vi "ke2002_init.vi"(8 "error in":errorcluster, 11 "VISA in":refnum<visa-resource-name>) -> (0 "error out":errorcluster, 2 "ID":string, 3 "VISA out":refnum<visa-resource-name>)   [LabVIEW 2020]
uses:
  <vilib>/Instr/_visa.llb/VISA GPIB Control REN Mode.ctl
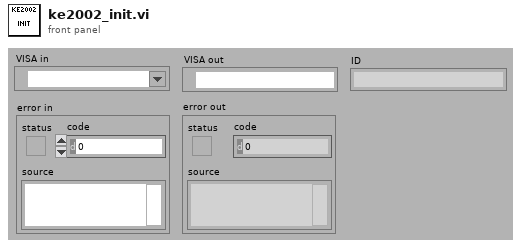
[diagram p1: front panel]
types:
  T1 = cluster{"Status":bool, "Code":i32, "Source (VI Name)":string}
  T2 = cluster{"error":bool, "code":i32, "source":string}
  T3 = typedef "VISA GPIB Control REN Mode.ctl" = u16
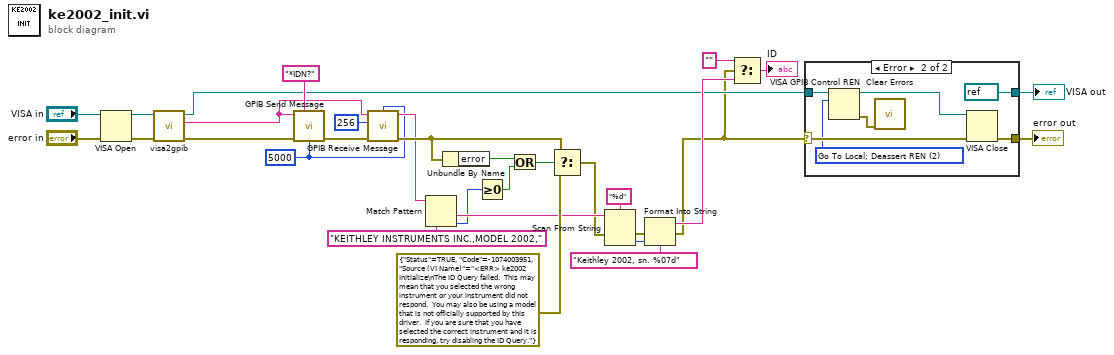
[diagram p0: block diagram]
diagram:
  w1 = u32 5000 ("timeout ms")
  n1 = VISA Open(error in (no error)="error in", VISA resource name="VISA in") -> (VISA resource name=w25:refnum<visa-resource-name>, error out=w26:errorcluster)  [unwired: 3 in]
  n2 = call "visa2gpib.vi"("error in"=w26, "VISA in"=w25) -> ("error out"=w24:errorcluster, "combined address"=w23:string, "VISA out"=w4:refnum<visa-resource-name>)  [unwired: 7 in]
  n3 = call "GPIB Send Message.vi"("timeout ms"=w1, "address string"=w23, "write buffer"="*IDN?", "error in"=w24) -> ("error out"=w31:T2)  [unwired: 3 in, 2 out]
  n4 = call "GPIB Receive Message.vi"("timeout ms"=w1, "address string"=w23, "byte count"=256, "error in"=w31) -> ("read buffer"=w17:string, "error out"=w19:T2)  [unwired: 3 in, 1 out]
  n5 = Match Pattern(string=w17, regular expression="KEITHLEY INSTRUMENTS INC.,MODEL 2002,") -> (after substring=w16:string, offset past match=w7:i32)  [unwired: 1 in, 2 out]
  n6 = Unbundle By Name(w19) -> ("error"=w21:bool)
  n7 = Greater Or Equal To 0?(x=w7) -> (x >= 0?=w6:bool)
  n8 = Or(x=w21, y=w6) -> (x .or. y?=w22:bool)
  n9 = Select(t=w19, s=w22, f=T1 {"Status"=TRUE, "Code"=-1074003951, "Source (VI Name)"="<ERR> ke2002 Initialize\nThe ID Query failed.  This may mean that you selected the wrong instrument or your instrument did not respond.  You may also be using a model that is not officially supported by this driver.  If you are sure that you have selected the correct instrument and it is responding, try disabling the ID Query."}) -> (s? t:f=w14:T1)
  n10 = Scan From String(format string="%d", input string=w16, error in=w14) -> (error out=w13:errorcluster, output 1=w12:i32)  [unwired: 2 in, 2 out]
  n11 = Format Into String(format string="Keithley 2002, sn. %07d", error in=w13, w12) -> (resulting string=w10:string, error out=w2:errorcluster)  [unwired: 1 in]
  n12 = Select(t="", s=w2, f=w10) -> (s? t:f=→"ID":string)
  n13 = case shown="Error" w2 {
    selector: w2 -> [w32 w38]
    tunnel: [w32 w40] -> w5
    tunnel: w4 -> [w33 w37]
    tunnel: [w33 refnum<visa-resource-name> refnum ("VISA out")] -> w3
    frame No Error {
    }
    frame Error {
      w35 = T3 2 items=["Deassert REN", "Assert REN", "Go To Local; Deassert REN ", "Assert REN; Address Device", "Local Lockout (Addressed Devices)", "Local Lockout (This Device)", "Go To Local"] ("Mode")
      n14 = VISA GPIB Control REN(10:w35, 11:w37) -> (0:w34:errorcluster, 3:w36:refnum<visa-resource-name>)  [unwired: 1 in]
      n15 = call <vilib>:"Clear Errors.vi"("error in (no error)"=w34) -> ()  [unwired: 5 in, 2 out]
      n16 = VISA Close(VISA resource name=w36, error in (no error)=w38) -> (error out=w40:errorcluster)
    }
  }
  "VISA out" <- w3
  "error out" <- w5
